vi "Map Channels (Single).vi"(8 "error in (no error)":errorcluster, 9 "Destination":string, 10 "Source":string, 11 "Loop Data":T1) -> (0 "error out":errorcluster)   [LabVIEW 2016, in "System Mapping Tool.lvlib"]
uses:
  System Mapping Tool.lvlib
  TypeDefs/Loop Data.ctl
  TypeDefs/UI Refs.ctl
  NationalInstruments.VeriStand.SystemDefinitionAPI
  NationalInstruments.VeriStand.SystemStorageUI
  Mapping Error Handler (Single).vi
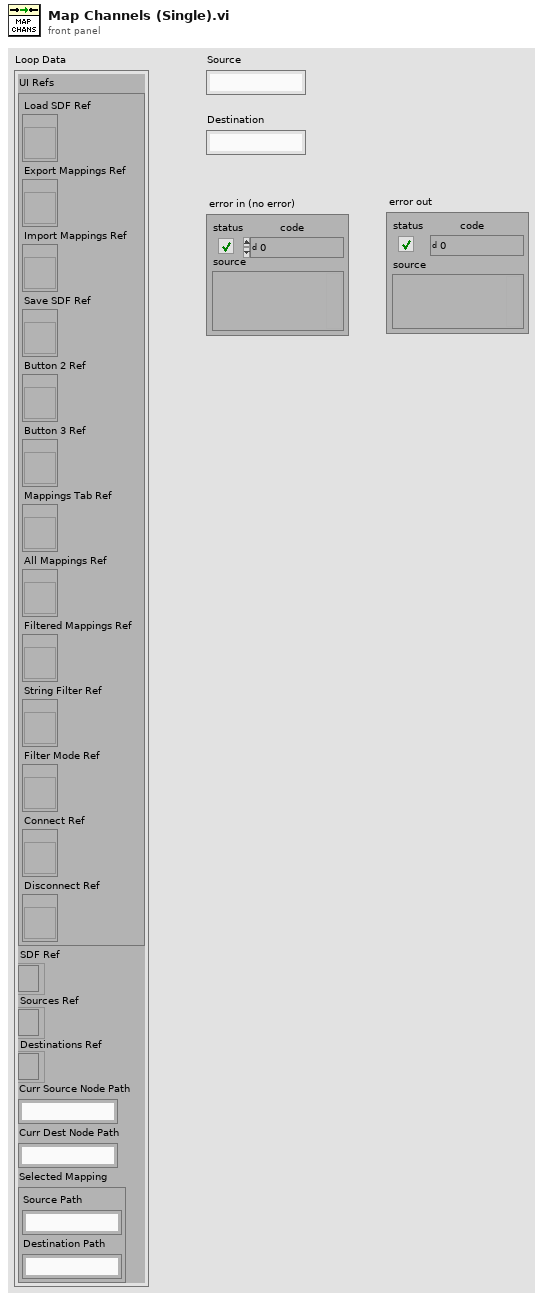
[diagram p1: front panel]
types:
  T1 = typedef "System Mapping Tool.lvlib/Loop Data.ctl" = cluster{"UI Refs":T2, "SDF Ref":refnum<k24>, "Sources Ref":refnum<k24>, "Destinations Ref":refnum<k24>, "Curr Source Node Path":string, "Curr Dest Node Path":string, "Selected Mapping":cluster{"Source Path":string, "Destination Path":string}}
  T2 = typedef "System Mapping Tool.lvlib/UI Refs.ctl" = cluster{"Load SDF Ref":refnum<vi>, "Export Mappings Ref":refnum<vi>, "Import Mappings Ref":refnum<vi>, "Save SDF Ref":refnum<vi>, "Button 2 Ref":refnum<vi>, "Button 3 Ref":refnum<vi>, "Mappings Tab Ref":refnum<vi>, "All Mappings Ref":refnum<vi>, "Filtered Mappings Ref":refnum<vi>, "String Filter Ref":refnum<vi>, "Filter Mode Ref":refnum<vi>, "Connect Ref":refnum<vi>, "Disconnect Ref":refnum<vi>}
  T3 = typedef "System Mapping Tool.lvlib/Mapping Error Cluster.ctl" = cluster{"Error?":bool, "Reason":T4, "Source":string, "Destination":string, "Line":i32}
  T4 = typedef "System Mapping Tool.lvlib/Mapping Error.ctl" = enum16{"No error", "Channels already mapped", "Source is not valid", "Destination is not valid", "Destination already mapped", "Destination mapped twice"}
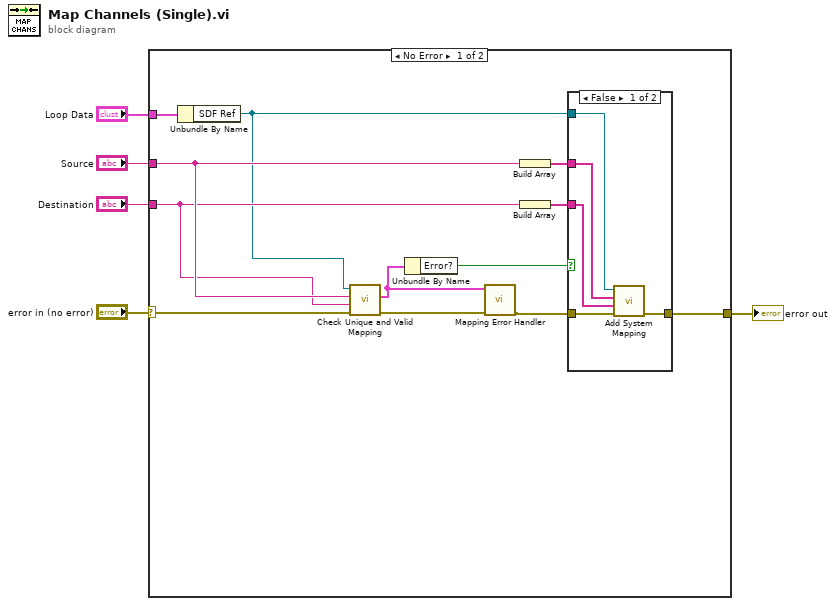
[diagram p0: block diagram]
diagram:
  n1 = case shown="No Error" "error in (no error)" {
    selector: "error in (no error)" -> [w17 w24]
    tunnel: [w16 w24] -> w4
    tunnel: "Source" -> [w14 _]
    tunnel: "Destination" -> [w13 _]
    tunnel: "Loop Data" -> [w15 _]
    frame No Error {
      n2 = Unbundle By Name(w15) -> ("SDF Ref"=w12:refnum<k24>)
      n3 = call "Check Unique and Valid Mapping.vi"("error in (no error)"=w17, "Destination Path"=w13, "Source Path"=w14, "SDF Ref"=w12) -> ("error out"=w8:errorcluster, "Mapping Error"=w6:T3)  [unwired: 6 in]
      n4 = Unbundle By Name(w6) -> ("Error?"=w11:bool)
      n5 = call-poly "Mapping Error Handler.vi"("error in (no error)"=w8, "Mapping Error"=w6) -> ("error out"=w7:errorcluster)  [unwired: 8 in, 1 out]
      n6 = Build Array(w14) -> (w9:string[])
      n7 = Build Array(w13) -> (w10:string[])
      n8 = case shown="False" w11 {
        tunnel: [w22 w23] -> w16
        tunnel: w7 -> [w21 w23]
        tunnel: w10 -> [w19 _]
        tunnel: w9 -> [w18 _]
        tunnel: w12 -> [w20 _]
        frame False {
          n9 = call "Add System Mapping.vi"("error in (no error)"=w21, "Destinations"=w19, "Sources"=w18, "SDF Ref"=w20) -> ("error out"=w22:errorcluster)  [unwired: 7 in]
        }
        frame True {
        }
      }
    }
    frame Error {
    }
  }
  "error out" <- w4
